vi "Configuration.vi"(6 "Return Data":refnum<user-event>, 8 "error in (no error)":errorcluster, 9 "Exit Running Config":refnum<user-event>, 10 "Panel in":refnum<class "Panel.lvclass">, 11 "Path Data Type in":refnum<class "Path Data Type.lvclass">) -> (0 "error out":errorcluster, 3 "Path Data Type out":refnum<class "Path Data Type.lvclass">)   [LabVIEW 2018, in "Path Data Type.lvclass"]
uses:
  Path Data Type.lvclass
  D:/Code/QControls Extended/DataGrid/DataGrid Configuration/Data Type Classes/Generic/Generic Data Type.lvclass
  <vilib>/MGI/Panel Manager/Panel/Panel/Panel.lvclass
  Generic/Generic Data Type.lvclass
  Files or Folders.ctl
  New or Existing.ctl
  Path Data Type.lvclass/Path Data Type.ctl
  Generic/Generic Data Type.lvclass/Generic Data Type.ctl
  Generic/Write Column Header.vi
  Generic/Read Column Header.vi
panel:
  in  "Main Tab":enum32{"Column Format", "Browse Options"}(tab)
  in  "Column Header":string
  in  "Default Value":path
  in  "TreatLLBsasfolders":bool
  in  "New or Existing":T1
  in  "Files or Folders":T2
  in  "Browse Button Options":T3(ring)
  in  "Prompt":string
  in  "Pattern":string
  in  "Start Path":path
  in  "Pattern Label":string
  in  "Button Text":string
  # "Path Column"
  # "Selection Mode"
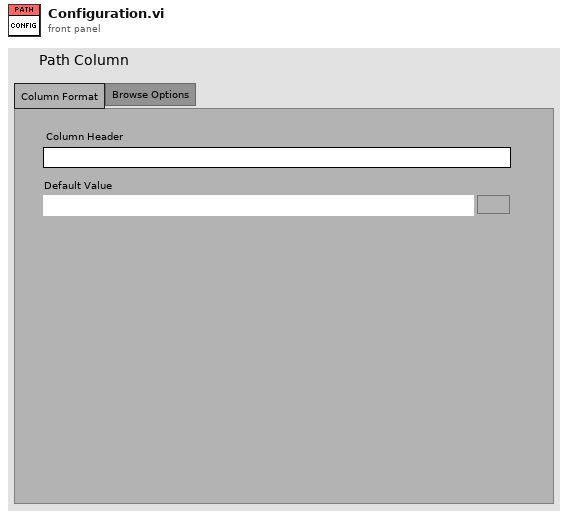
[diagram p1: front panel]
types:
  T1 = typedef "Path Data Type.lvclass/New or Existing.ctl" = enum32{"Existing", "New", "New or Existing"}
  T2 = typedef "Path Data Type.lvclass/Files or Folders.ctl" = enum32{"Files", "Folders", "Files or Folders"}
  T3 = enum16{"Enabled", "Disabled", "Disabled and Grayed Out", "Not Visible"}
  T4 = typedef "Path Data Type.lvclass/Selection Mode.ctl" = enum32{"existing file", "new file", "new or existing file", "existing dir", "new dir", "new or existing dir", "existing file (use LLBs)", "new file (use LLBs)", "new or existing file (use LLBs)", "new or existing file or directory (use LLBs)", "existing dir (use LLBs)", "new dir (use LLBs)", "new or existing dir (use LLBs)", "existing file or dir", "new file or dir", "new or existing file or dir", "existing file or dir (use LLBs)", "new file or dir (use LLBs)"}
  T5 = enum8{"Enabled", "Disabled", "Disabled and Grayed Out"}
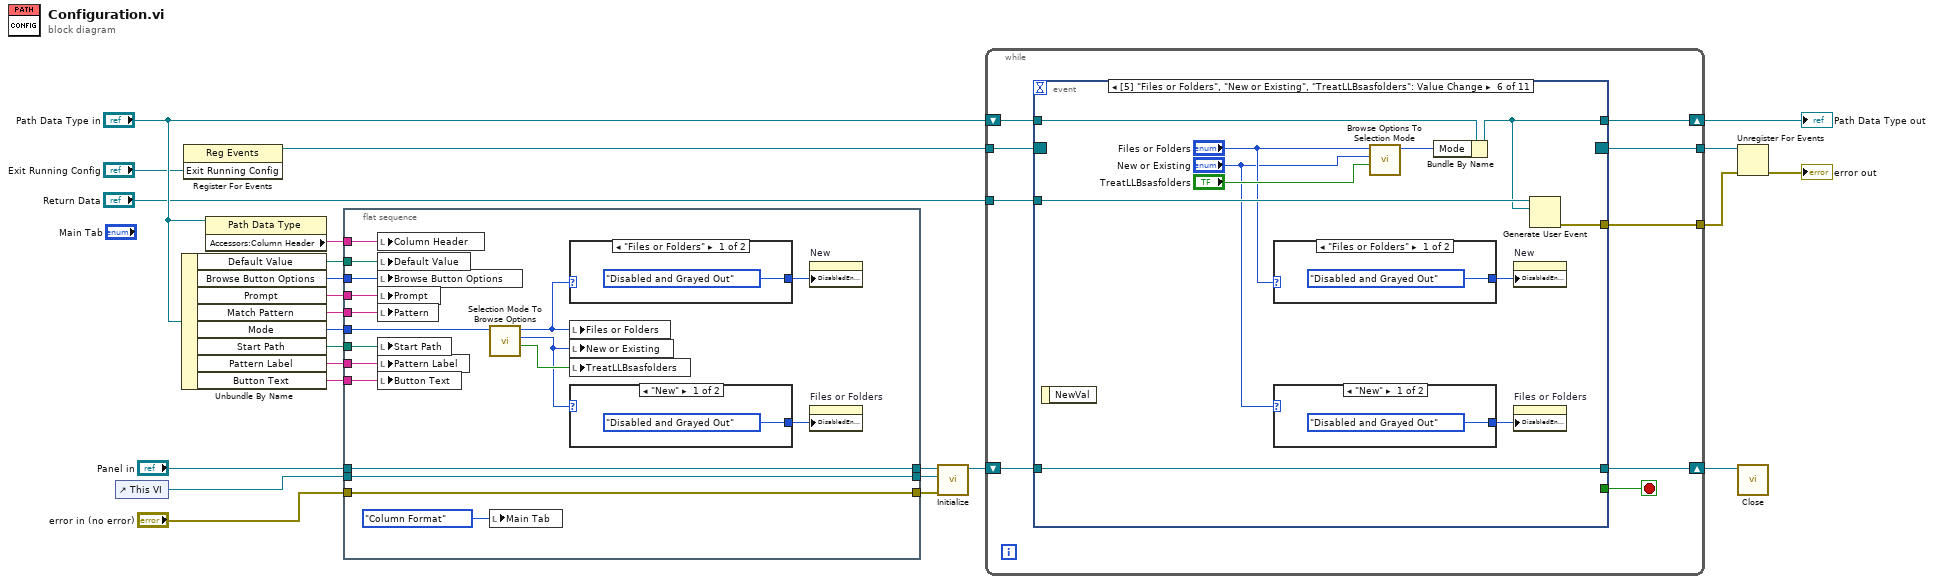
[diagram p0: block diagram]
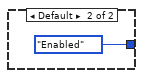
[diagram p2: hidden frame]
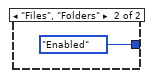
[diagram p3: hidden frame]
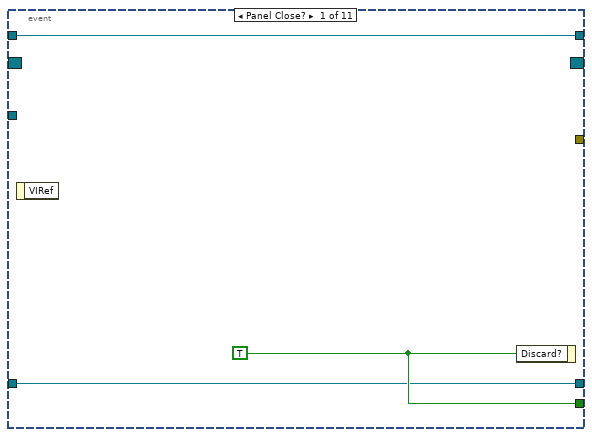
[diagram p4: hidden frame]
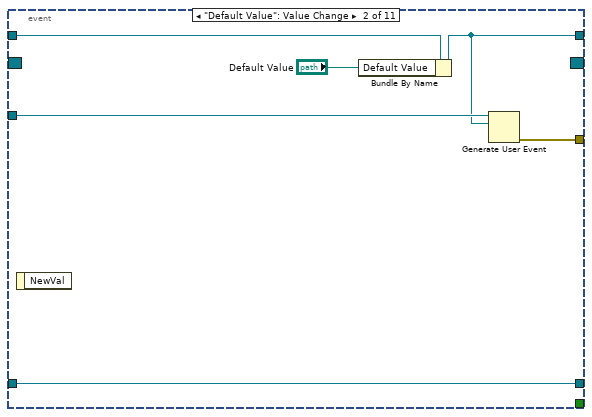
[diagram p5: hidden frame]
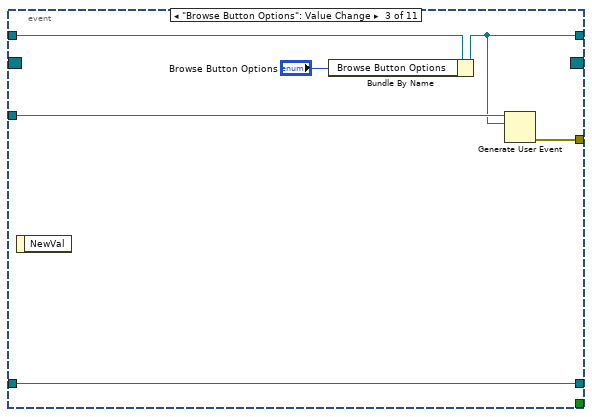
[diagram p6: hidden frame]
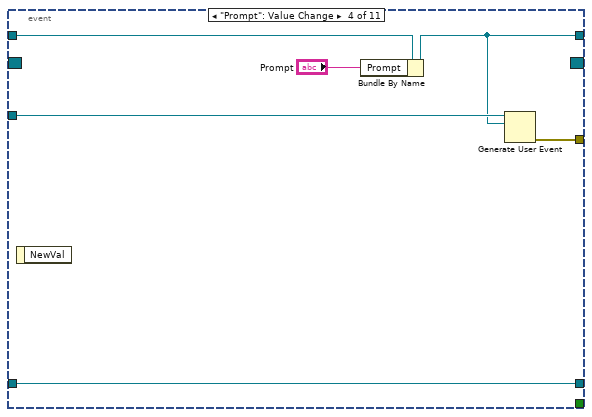
[diagram p7: hidden frame]
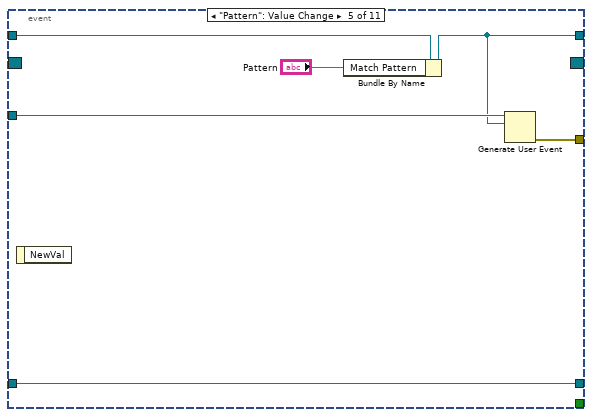
[diagram p8: hidden frame]
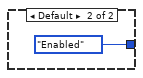
[diagram p9: hidden frame]
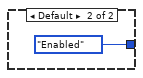
[diagram p10: hidden frame]
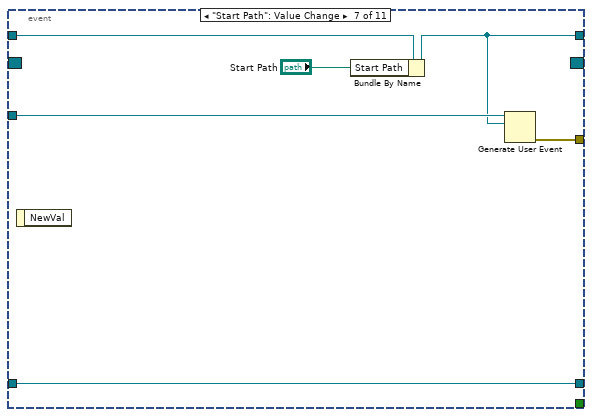
[diagram p11: hidden frame]
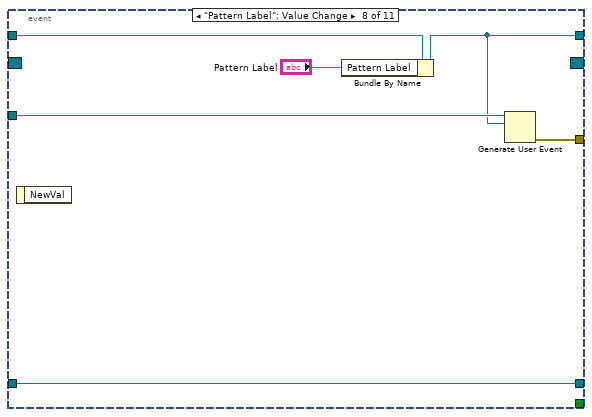
[diagram p12: hidden frame]
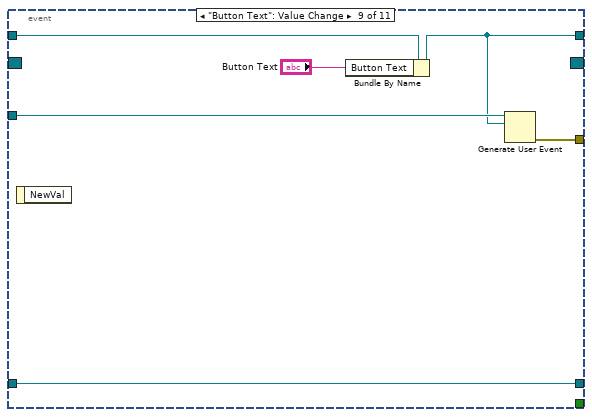
[diagram p13: hidden frame]
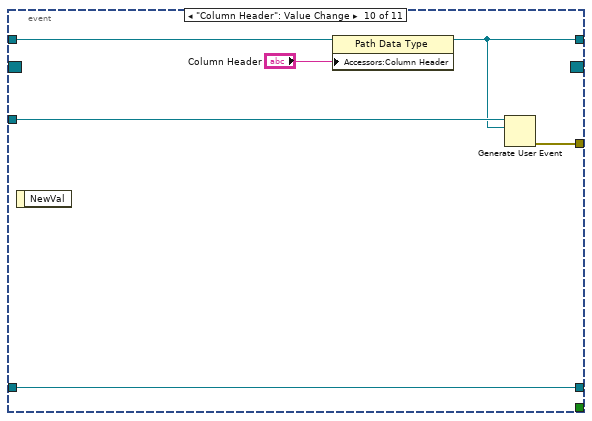
[diagram p14: hidden frame]
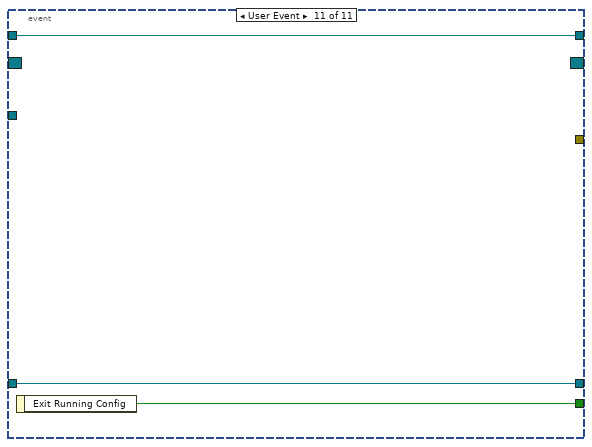
[diagram p15: hidden frame]
diagram:
  n1 = control-ref of="This VI"() -> (w9:refnum<vi>)
  n2 = Unbundle By Name("Path Data Type in") -> ("Default Value"=w24:path, "Browse Button Options"=w11:T3, "Prompt"=w6:string, "Match Pattern"=w5:string, "Mode"=w4:T4, "Start Path"=w3:path, "Pattern Label"=w2:string, "Button Text"=w1:string)
  n3 = register-events("Exit Running Config") -> (reference out=w17:refnum<event-registration>)  [unwired: 2 in, 1 out]
  n4 = property class="Path Data Type"(reference="Path Data Type in") -> ("Accessors:Column Header"=w25:string)  [unwired: 1 in, 2 out]
  n5 = flat-sequence {
    tunnel: w11 -> [w43]
    tunnel: "Panel in" -> [w42]
    tunnel: [w42] -> w20
    tunnel: [w41] -> w21
    tunnel: w9 -> [w41]
    tunnel: "error in (no error)" -> [w40]
    tunnel: [w40] -> w23
    tunnel: w24 -> [w39]
    tunnel: w25 -> [w38]
    tunnel: w6 -> [w37]
    tunnel: w5 -> [w36]
    tunnel: w4 -> [w32]
    tunnel: w3 -> [w35]
    tunnel: w2 -> [w34]
    tunnel: w1 -> [w33]
    frame #0 {
      n6 = local write "Column Header"(w38) -> ()
      n7 = local write "Default Value"(w39) -> ()
      n8 = local write "Browse Button Options"(w43) -> ()
      n9 = local write "Prompt"(w37) -> ()
      n10 = local write "Pattern"(w36) -> ()
      n11 = local write "Start Path"(w35) -> ()
      n12 = local write "Pattern Label"(w34) -> ()
      n13 = local write "Button Text"(w33) -> ()
      n14 = call "Selection Mode To Browse Options.vi"("Selection Mode"=w32) -> ("Treat LLB's as Folders"=w31:bool, "New or Existing"=w28:T1, "Files or Folders"=w30:T2)  [unwired: 8 in]
      n15 = local write "Main Tab"(enum32{"Column Format", "Browse Options"}."Column Format" ("Main Tab")) -> ()
      n16 = case shown="\"Files or Folders\"" w30 {
        tunnel: [T5."Disabled and Grayed Out" ("Disabled") T5."Enabled" ("Disabled")] -> w29
        frame "Files or Folders" {
        }
        frame "Files", "Folders" {
        }
      }
      n17 = local write "Files or Folders"(w30) -> ()
      n18 = local write "New or Existing"(w28) -> ()
      n19 = local write "TreatLLBsasfolders"(w31) -> ()
      n20 = case shown="\"New\"" w28 {
        tunnel: [T5."Disabled and Grayed Out" ("Disabled") T5."Enabled" ("Disabled")] -> w27
        frame "New" {
        }
        frame Default {
        }
      }
      n21 = property on="New" class="Bool (strict)"("DisabledEnum"=w29) -> ()  [unwired: 2 in, 2 out]
      n22 = property on="Files or Folders" class="Bool (strict)"("DisabledEnum"=w27) -> ()  [unwired: 2 in, 2 out]
    }
  }
  n23 = call <vilib>:"Initialize.vi"("error in (no error)"=w23, "VI Refnum"=w21, "Panel In"=w20) -> ("Panel Out"=w19:refnum<class "Panel.lvclass">)  [unwired: 6 in, 2 out]
  n24 = while {
    shift-right: [w50] -> w14
    shift-left: "Path Data Type in" -> [w56]
    shift-right: [w52] -> w18
    shift-left: w19 -> [w53]
    tunnel: w17 -> [w54]
    tunnel: [w51] -> w16
    tunnel: "Return Data" -> [w49]
    tunnel: [w48] -> w22
    stop <- w55 stop-if-true
    n25 = event shown="[5] \"Files or Folders\", \"New or Existing\", \"TreatLLBsasfolders\": Value Change" {
      selector: w54 -> [_ _ _ _ _ _ _ _ _ _ _]
      dyn-events: [_ _ _ _ _ _ _ _ _ _ _] -> w51
      timeout: _ -> [_ _ _ _ _ _ _ _ _ _ _]
      tunnel: w56 -> [w59 w64 w70 w76 w82 w93 w103 w109 w115 w119 w125]
      tunnel: [w59 w62 w68 w74 w80 w91 w101 w107 w113 w118 w125] -> w50
      tunnel: [w58 _ _ _ _ _ _ _ _ _ w124] -> w55
      tunnel: w53 -> [w57 w65 w71 w77 w83 w94 w104 w110 w116 w122 w123]
      tunnel: [w57 w65 w71 w77 w83 w94 w104 w110 w116 w122 w123] -> w52
      tunnel: w49 -> [_ w63 w69 w75 w81 w92 w102 w108 w114 w121 _]
      tunnel: [_ w61 w67 w73 w79 w90 w100 w106 w112 w120 _] -> w48
      event Panel Close? {
        w58 = TRUE
        n26 = event-data() -> ()  [unwired: 1 in, 1 out]
        n27 = event-data("Discard?"=w58) -> ()  [unwired: 1 in, 1 out]
      }
      event "Default Value": Value Change {
        n28 = event-data() -> ()  [unwired: 1 in, 1 out]
        n29 = Bundle By Name(cluster=w64, "Default Value"="Default Value") -> (w62:refnum<class "Path Data Type.lvclass">)
        n30 = Generate User Event(user event=w63, event data cluster=w62) -> (error out=w61:errorcluster)  [unwired: 2 in, 1 out]
      }
      event "Browse Button Options": Value Change {
        n31 = event-data() -> ()  [unwired: 1 in, 1 out]
        n32 = Bundle By Name(cluster=w70, "Browse Button Options"="Browse Button Options") -> (w68:refnum<class "Path Data Type.lvclass">)
        n33 = Generate User Event(user event=w69, event data cluster=w68) -> (error out=w67:errorcluster)  [unwired: 2 in, 1 out]
      }
      event "Prompt": Value Change {
        n34 = event-data() -> ()  [unwired: 1 in, 1 out]
        n35 = Bundle By Name(cluster=w76, "Prompt"="Prompt") -> (w74:refnum<class "Path Data Type.lvclass">)
        n36 = Generate User Event(user event=w75, event data cluster=w74) -> (error out=w73:errorcluster)  [unwired: 2 in, 1 out]
      }
      event "Pattern": Value Change {
        n37 = event-data() -> ()  [unwired: 1 in, 1 out]
        n38 = Bundle By Name(cluster=w82, "Match Pattern"="Pattern") -> (w80:refnum<class "Path Data Type.lvclass">)
        n39 = Generate User Event(user event=w81, event data cluster=w80) -> (error out=w79:errorcluster)  [unwired: 2 in, 1 out]
      }
      event "TreatLLBsasfolders": Value Change {
        n40 = event-data() -> ()  [unwired: 1 in, 1 out]
        n41 = case shown="\"Files or Folders\"" "Files or Folders" {
          tunnel: [T5."Disabled and Grayed Out" ("Disabled") T5."Enabled" ("Disabled")] -> w87
          frame "Files or Folders" {
          }
          frame Default {
          }
        }
        n42 = case shown="\"New\"" "New or Existing" {
          tunnel: [T5."Disabled and Grayed Out" ("Disabled") T5."Enabled" ("Disabled")] -> w85
          frame "New" {
          }
          frame Default {
          }
        }
        n43 = call "Browse Options To Selection Mode.vi"("Treat LLB's as Folders"="TreatLLBsasfolders", "New or Existing"="New or Existing", "Files or Folders"="Files or Folders") -> ("Selection Mode"=w89:T4)  [unwired: 8 in]
        n44 = Bundle By Name(cluster=w93, "Mode"=w89) -> (w91:refnum<class "Path Data Type.lvclass">)
        n45 = property on="New" class="Bool (strict)"("DisabledEnum"=w87) -> ()  [unwired: 2 in, 2 out]
        n46 = property on="Files or Folders" class="Bool (strict)"("DisabledEnum"=w85) -> ()  [unwired: 2 in, 2 out]
        n47 = Generate User Event(user event=w92, event data cluster=w91) -> (error out=w90:errorcluster)  [unwired: 2 in, 1 out]
      }
      event "Start Path": Value Change {
        n48 = event-data() -> ()  [unwired: 1 in, 1 out]
        n49 = Bundle By Name(cluster=w103, "Start Path"="Start Path") -> (w101:refnum<class "Path Data Type.lvclass">)
        n50 = Generate User Event(user event=w102, event data cluster=w101) -> (error out=w100:errorcluster)  [unwired: 2 in, 1 out]
      }
      event "Pattern Label": Value Change {
        n51 = event-data() -> ()  [unwired: 1 in, 1 out]
        n52 = Bundle By Name(cluster=w109, "Pattern Label"="Pattern Label") -> (w107:refnum<class "Path Data Type.lvclass">)
        n53 = Generate User Event(user event=w108, event data cluster=w107) -> (error out=w106:errorcluster)  [unwired: 2 in, 1 out]
      }
      event "Button Text": Value Change {
        n54 = event-data() -> ()  [unwired: 1 in, 1 out]
        n55 = Bundle By Name(cluster=w115, "Button Text"="Button Text") -> (w113:refnum<class "Path Data Type.lvclass">)
        n56 = Generate User Event(user event=w114, event data cluster=w113) -> (error out=w112:errorcluster)  [unwired: 2 in, 1 out]
      }
      event "Column Header": Value Change {
        n57 = event-data() -> ()  [unwired: 1 in, 1 out]
        n58 = property class="Path Data Type"(reference=w119, "Accessors:Column Header"="Column Header") -> (reference out=w118:refnum<class "Path Data Type.lvclass">)  [unwired: 1 in, 1 out]
        n59 = Generate User Event(user event=w121, event data cluster=w118) -> (error out=w120:errorcluster)  [unwired: 2 in, 1 out]
      }
      event User Event {
        n60 = event-data() -> ("Exit Running Config"=w124:bool)  [unwired: 1 in]
      }
    }
  }
  "Path Data Type out" <- w14
  n61 = Unregister For Events(event registration refnum=w16, error in=w22) -> (error out=→"error out":errorcluster)
  n62 = call-dynamic "Close.vi"("Panel In"=w18) -> ()  [unwired: 10 in, 1 out]
